vi "Close_FP.vi"(8 "error in (no error)":errorcluster, 11 "VI path":path) -> (0 "error out":errorcluster)   [LabVIEW 2019]
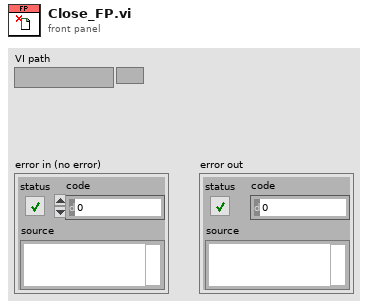
[diagram p1: front panel]
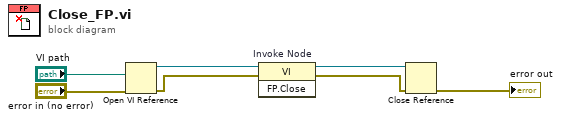
[diagram p0: block diagram]
diagram:
  n1 = Open VI Reference(vi path="VI path", error in (no error)="error in (no error)") -> (vi reference=w4:refnum<vi>, error out=w5:errorcluster)  [unwired: 4 in]
  n2 = invoke on="Invoke Node" class="VI" method="FP.Close"(reference=w4, error in=w5) -> (reference out=w3:refnum<vi>, error out=w2:errorcluster)  [unwired: 1 in, 1 out]
  n3 = Close Reference(reference=w3, error in (no error)=w2) -> (error out=→"error out":errorcluster)
